vi "mod_Create MSK Sync Param.vi"(0 "TSC":u16(ring) items=["0", "1", "2", "3", "4", "5", "6", "7"], 5 "MSK System Parameters":T1={"differential encoding enable"=enum."enable", "samples per symbol (16)"=16}, 7 "Sync Indent, symbols":i32=61, 9 "user bits":i8[](array[numeric]), 11 "error in (no error)":errorcluster) -> (4 "Synchronization Parameters":T2 {"Sync Sequence" format="%.2f"}, 15 "error out":errorcluster)   [LabVIEW 2020, in "niDMT.lvlib"]
uses:
  <vilib>/addons/Modulation/niDMT.lvlib
  <vilib>/addons/Modulation/Digital/Support/Controls/MSK System Parameters.ctl
  <vilib>/addons/Modulation/Digital/General/MT Map Bits to MSK symbols.vi
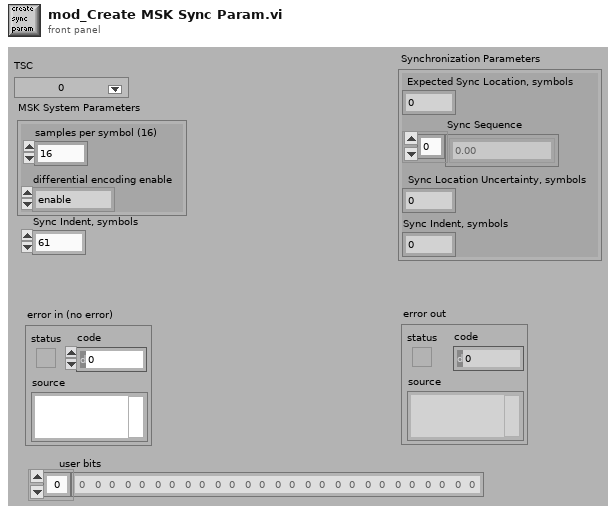
[diagram p1: front panel]
types:
  T1 = typedef "niDMT.lvlib/MSK System Parameters.ctl" = cluster{"differential encoding enable":enum16{"disable", "enable"}, "samples per symbol (16)":i32}
  T2 = cluster{"Expected Sync Location, symbols":i32, "Sync Sequence":cdb[], "Sync Location Uncertainty, symbols":i32, "Sync Indent, symbols":i32}
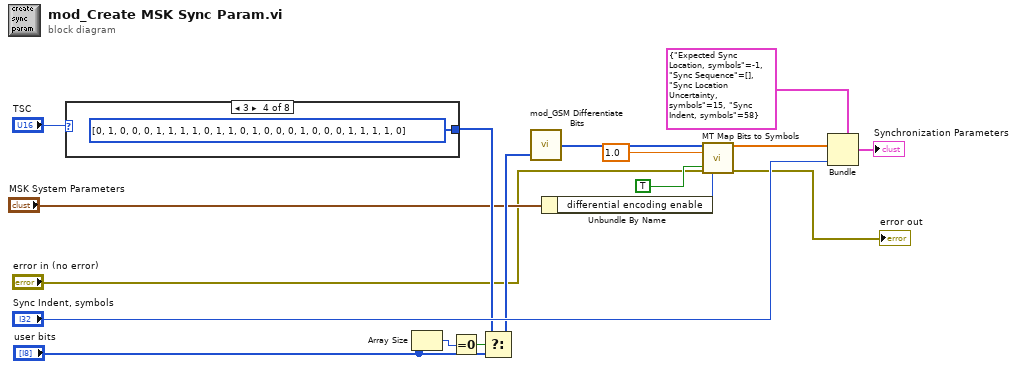
[diagram p0: block diagram]
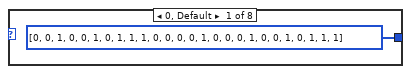
[diagram p2: hidden frame]
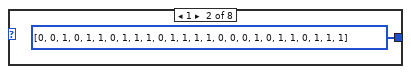
[diagram p3: hidden frame]
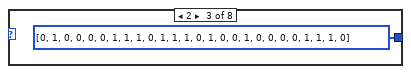
[diagram p4: hidden frame]
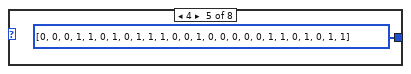
[diagram p5: hidden frame]
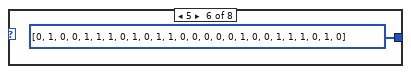
[diagram p6: hidden frame]
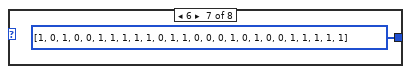
[diagram p7: hidden frame]
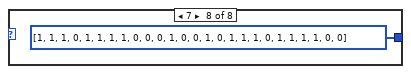
[diagram p8: hidden frame]
diagram:
  n1 = case shown="3" "TSC" {
    tunnel: [i8[] [0, 0, 1, 0, 0, 1, 0, 1, 1, 1, 0, 0, 0, 0, 1, 0, 0, 0, 1, 0, 0, 1, 0, 1, 1, 1] i8[] [0, 0, 1, 0, 1, 1, 0, 1, 1, 1, 0, 1, 1, 1, 1, 0, 0, 0, 1, 0, 1, 1, 0, 1, 1, 1] i8[] [0, 1, 0, 0, 0, 0, 1, 1, 1, 0, 1, 1, 1, 0, 1, 0, 0, 1, 0, 0, 0, 0, 1, 1, 1, 0] i8[] [0, 1, 0, 0, 0, 1, 1, 1, 1, 0, 1, 1, 0, 1, 0, 0, 0, 1, 0, 0, 0, 1, 1, 1, 1, 0] i8[] [0, 0, 0, 1, 1, 0, 1, 0, 1, 1, 1, 0, 0, 1, 0, 0, 0, 0, 0, 1, 1, 0, 1, 0, 1, 1] i8[] [0, 1, 0, 0, 1, 1, 1, 0, 1, 0, 1, 1, 0, 0, 0, 0, 0, 1, 0, 0, 1, 1, 1, 0, 1, 0] i8[] [1, 0, 1, 0, 0, 1, 1, 1, 1, 1, 0, 1, 1, 0, 0, 0, 1, 0, 1, 0, 0, 1, 1, 1, 1, 1] i8[] [1, 1, 1, 0, 1, 1, 1, 1, 0, 0, 0, 1, 0, 0, 1, 0, 1, 1, 1, 0, 1, 1, 1, 1, 0, 0]] -> w13
    frame 0, Default {
    }
    frame 1 {
    }
    frame 2 {
    }
    frame 3 {
    }
    frame 4 {
    }
    frame 5 {
    }
    frame 6 {
    }
    frame 7 {
    }
  }
  n2 = Array Size(array="user bits") -> (size(s)=w12:i32)
  n3 = Equal To 0?(x=w12) -> (x = 0?=w11:bool)
  n4 = Select(t=w13, s=w11, f="user bits") -> (s? t:f=w9:i8[])
  n5 = call <vilib>:"mod_GSM Differentiate Bits.vi"("bits in"=w9) -> ("diffed bits"=w8:i8[])  [unwired: 1 in]
  n6 = Unbundle By Name("MSK System Parameters") -> ("differential encoding enable"=w3:enum16{"disable", "enable"})
  n7 = call-poly <vilib>:"MT Map Bits to Symbols.vi"("input bit stream"=w8, "symbol rate, Hz"=1.0 ("Symbol Rate, Hz"), "error in (no error)"="error in (no error)", "differential encoding enable"=w3, "reset? (T)"=TRUE ("Reset")) -> ("symbols"=w5:dbl[], "error out"=→"error out":errorcluster)  [unwired: 9 out]
  n8 = Bundle(cluster=T2 {"Expected Sync Location, symbols"=-1, "Sync Sequence"=[], "Sync Location Uncertainty, symbols"=15, "Sync Indent, symbols"=58} ("Synchronization Parameters"), "Sync Sequence"=w5, "Sync Indent, symbols"="Sync Indent, symbols") -> (→"Synchronization Parameters":T2)  [unwired: 2 out]
